vi "Available Registers FG.vi"(6 "Action":T3, 8 "error in (no error)":errorcluster, 10 "Available Registers":T1[](array[typedef]) {"Data Type" format="%.0x"}, 11 "Item Ref":T4 format="%.0x") -> (0 "error out":errorcluster, 2 "Available Registers":T1[](array[typedef]) {"Data Type" format="%.0x"}, 3 "Item Ref out":T4=18446744073709551615 format="%.0x")   [LabVIEW 2019, in "FPGA Addon Shared.lvlib"]
uses:
  FPGA Addon Shared.lvlib
  Register Information.ctl
  Data Type.ctl
  <vilib>/NI VeriStand/Custom Device API/Custom Device Item Ref.ctl
  FG Action.ctl
  Constants.vi
  <vilib>/NI/NI VeriStand Advanced SysDef API/_SubVIs/SysDef.Property.Get.Variant.vi
  <vilib>/NI/NI VeriStand Advanced SysDef API/_SubVIs/SysDef.Property.Set.Variant.vi
  <vilib>/NI/NI VeriStand Advanced SysDef API/SysDef API/Advanced System Definition.lvlib
  <vilib>/NI VeriStand/Custom Device API/Custom Device API.lvlib
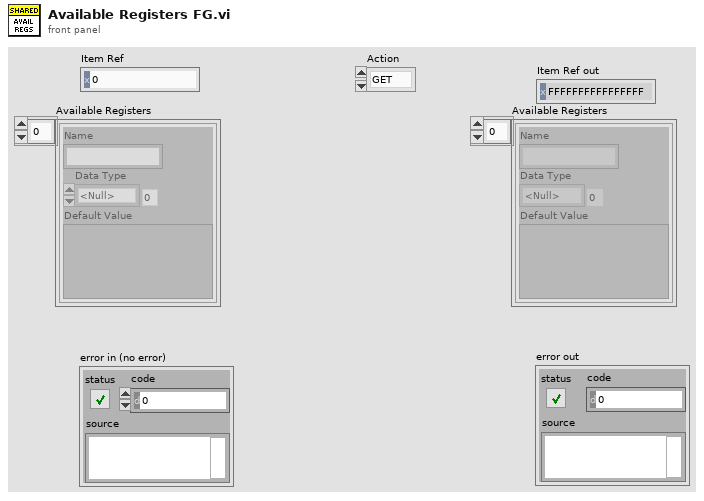
[diagram p1: front panel]
types:
  T1 = typedef "FPGA Addon Shared.lvlib/Register Information.ctl" = cluster{"Name":string, "Data Type":T2, "Default Value":variant}
  T2 = typedef "FPGA Addon Shared.lvlib/Data Type.ctl" = enum8{"<Null>", "I8", "I16", "I32", "I64", "U8", "U16", "U32", "U64", "SGL", "Boolean", "Analog PWM In Settings", "Analog PWM In", "Digital PWM In Settings", "Digital PWM In", "Digital PWM Out", "Sine Out", "FXP+/-24.5", "FXP+/-16.5", "FXP+/-32.8", "FXP+/-64.32", "FXP+/-16.7", "FXP+/-20.5", "FXP+/-27.5", "FXP+/-32.16", "FXP +16.3", "FXP +18.3", "Digital Static In", "Digital Static Out", "Digital Static In Settings", "Digital WSS Out", "Quad Encoder Settings", "Quad Encoder In"}
  T3 = typedef "FPGA Addon Shared.lvlib/FG Action.ctl" = enum8{"GET", "SET"}
  T4 = typedef "Custom Device API.lvlib/Custom Device Item Ref.ctl" = u64
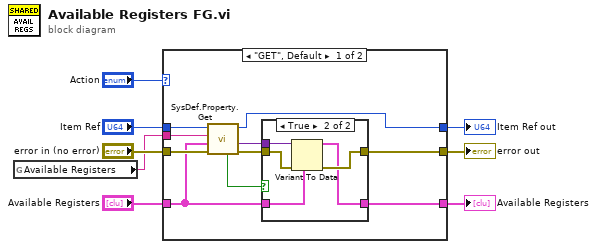
[diagram p0: block diagram]
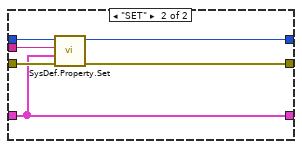
[diagram p3: hidden frame]
diagram:
  n1 = global read "Constants.vi" "Available Registers"() -> (w2:string)
  n2 = case shown="\"GET\", Default" "Action" {
    tunnel: "error in (no error)" -> [w18 w31]
    tunnel: "Item Ref" -> [w17 w30]
    tunnel: "Available Registers" -> [w15 w27]
    tunnel: [w13 w29] -> w8
    tunnel: [w10 w28] -> w4
    tunnel: [w11 w27] -> w1
    tunnel: w2 -> [w9 w26]
    frame "GET", Default {
      n3 = call-poly <vilib>:"SysDef.Property.Get.vi"("error in (no error)"=w18, "Value"=w15, "Property Name"=w9, "nodeID"=w17) -> ("error out"=w14:errorcluster, "Value"=w16:variant, "nodeID out"=w10:u64, "Found?"=w12:bool)  [unwired: 4 in]
      n4 = case shown="True" w12 {
        tunnel: w16 -> [_ w25]
        tunnel: w15 -> [w19 w24]
        tunnel: w14 -> [w20 w23]
        tunnel: [w20 w22] -> w13
        tunnel: [w19 w21] -> w11
        frame False {
        }
        frame True {
          n5 = Variant To Data(error in=w23, type=w24, Variant=w25) -> (data=w21:T1[], error out=w22:errorcluster)
        }
      }
    }
    frame "SET" {
      n6 = call-poly <vilib>:"SysDef.Property.Set.vi"("error in (no error)"=w31, "Value"=w27, "Property Name"=w26, "nodeID"=w30) -> ("error out"=w29:errorcluster, "nodeID out"=w28:u64)  [unwired: 6 in]
    }
  }
  "error out" <- w8
  "Item Ref out" <- w4
  "Available Registers" <- w1
